vi "solar_app Explore.vi"(8 "error in (no error)":errorcluster, 10 "Open Folder? (F)":bool, 11 "File or Folder Path":path) -> (0 "error out":errorcluster)   [LabVIEW 2018]
doc: "This VI opens a file or folder in windows explorer."
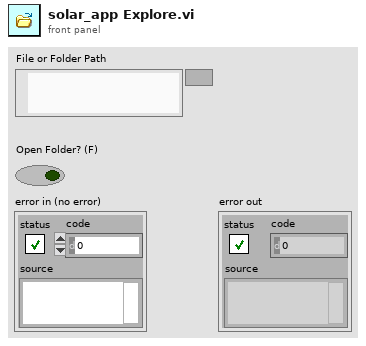
[diagram p1: front panel]
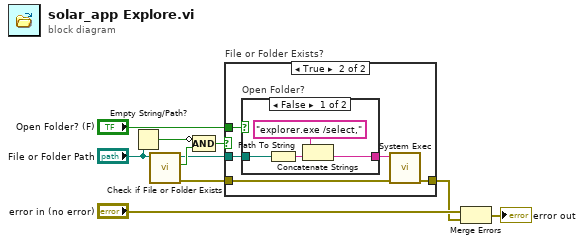
[diagram p0: block diagram]
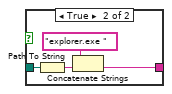
[diagram p3: hidden frame]
diagram:
  n1 = Empty String/Path?(string/path="File or Folder Path") -> (empty?=w8:bool)
  n2 = call <vilib>:"Check if File or Folder Exists.vi"("path"="File or Folder Path") -> ("error out"=w3:errorcluster, "file or folder exists?"=w7:bool, "dup path"=w6:path)  [unwired: 8 in]
  n3 = Compound Arithmetic op=AND(invert w8, w7) -> (w5:bool)
  n4 = case "File or Folder Exists?" shown="True" w5 {
    tunnel: w6 -> [_ w16]
    tunnel: "Open Folder? (F)" -> [_ w15]
    tunnel: w3 -> [w11 w13]
    tunnel: [w11 w12] -> w1
    frame False {
    }
    frame True {
      n5 = case "Open Folder?" shown="False" w15 {
        tunnel: w16 -> [w18 w22]
        tunnel: [w17 w21] -> w14
        frame False {
          n6 = Path To String(path=w18) -> (string=w19:string)
          n7 = Concatenate Strings("explorer.exe /select,", w19) -> (w17:string)
        }
        frame True {
          n8 = Path To String(path=w22) -> (string=w23:string)
          n9 = Concatenate Strings("explorer.exe ", w23) -> (w21:string)
        }
      }
      n10 = call <vilib>:"System Exec.vi"("error in (no error)"=w13, "command line"=w14) -> ("error out"=w12:errorcluster)  [unwired: 6 in, 3 out]
    }
  }
  n11 = Merge Errors("error in (no error)", w1) -> (→"error out":errorcluster)
